vi "Pre Launch Init.vi"(11 "Car Wash Controller in":refnum<class "Sim Entry Console Actor.lvclass">) -> (0 "error out":errorcluster, 3 "Car Wash Controller out":refnum<class "Sim Entry Console Actor.lvclass">)   [LabVIEW 2019, in "Sim Entry Console Actor.lvlib" / "Sim Entry Console Actor.lvclass"]
doc: "(<B>Filename</B>: Actor Framework.lvlib:Actor.lvclass:Pre Launch Init.vi)\n\nDefines behavior that occurs after the Launch Nested Actor method is invoked but before the actor's Actor Core method begins running.\n\nBy default, this method does nothing. A descendant class may override it to define behavior."
uses:
  Sim Entry Console Actor.lvclass
  Sim Entry Console Actor.lvclass/Sim Entry Console Actor.ctl
  Entry Console Actor/Entry Console Actor/Entry Console Actor.lvclass
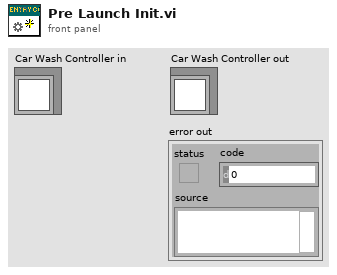
[diagram p1: front panel]
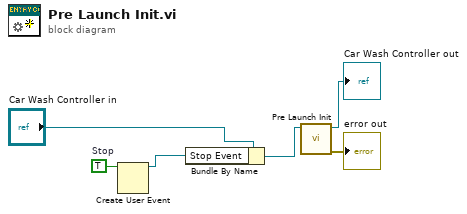
[diagram p0: block diagram]
diagram:
  w4 = TRUE  # Stop
  n1 = Create User Event(user event datatype=w4) -> (user event=w2:refnum<user-event>)  [unwired: 1 in, 1 out]
  n2 = Bundle By Name(cluster="Car Wash Controller in", "Stop Event"=w2) -> (w1:refnum<class "Sim Entry Console Actor.lvclass">)
  n3 = call-parent "Pre Launch Init.vi"("Actor in"=w1) -> ("error out"=→"error out":errorcluster, "Actor out"=→"Car Wash Controller out":refnum<class "Sim Entry Console Actor.lvclass">)  [unwired: 9 in]
